vi "Miniquads.IDQuery.vi"(0 "i ref in":refnum<vi>, 3 "ms timeout (10000)":i32=10000, 5 "error in (no error)":errorcluster) -> (14 "i ref out":refnum<vi>, 15 "DeviceID":string, 17 "timed out":bool, 19 "error out":errorcluster)   [LabVIEW 2014, in "Miniquads.lvlib"]
doc: "Gets and sets the device ID."
uses:
  Miniquads.lvlib
  CS_Core/CSSystem/CSSystemLib/CSSystemLib.lvlib
  CSlibraries-extern/DimLVEvent/NodeMon-LV/LVNodeInfo/LVNodeInfo.lvlib
  CS_Core/CSApplicationBaseClasses/DeviceBase/DeviceBase.lvlib
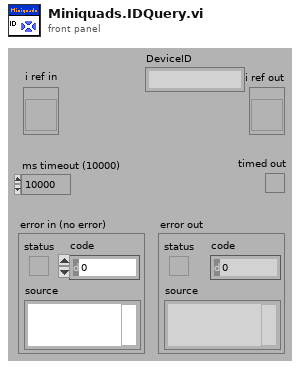
[diagram p1: front panel]
types:
  T1 = cluster{"Major":u16, "Minor":u16, "Fix":u16, "Build":u16}
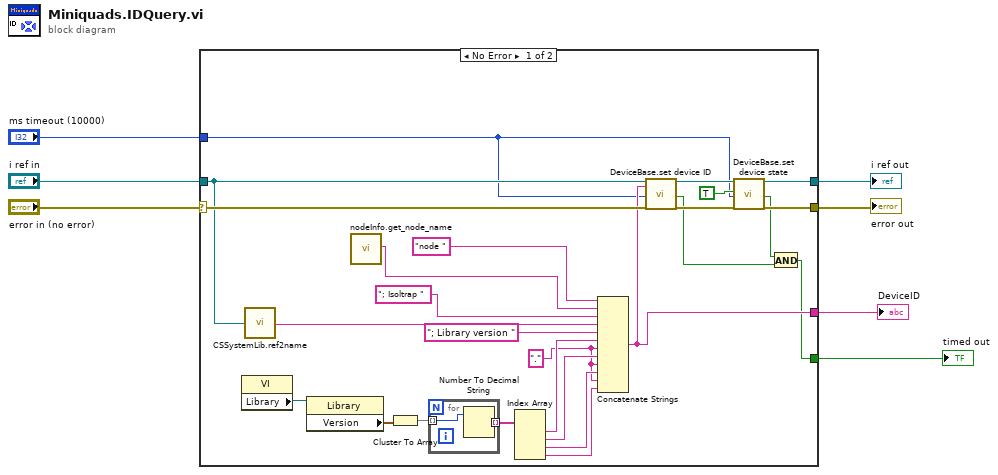
[diagram p0: block diagram]
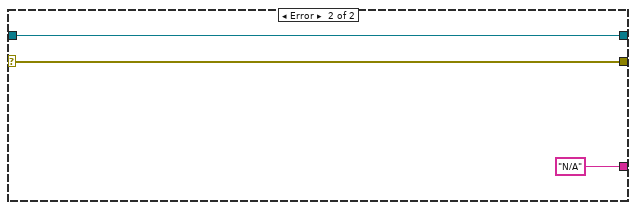
[diagram p2: hidden frame]
diagram:
  n1 = case shown="No Error" "error in (no error)" {
    selector: "error in (no error)" -> [w30 w37]
    tunnel: "i ref in" -> [w22 w38]
    tunnel: [w31 w38] -> w6
    tunnel: [w28 w37] -> w5
    tunnel: "ms timeout (10000)" -> [w11 _]
    tunnel: [w23 "N/A"] -> w2
    tunnel: [w8 _] -> w1
    frame No Error {
      w12 = "."
      n2 = property class="VI"() -> ("Library"=w21:refnum<vi>)  [unwired: 2 in, 2 out]
      n3 = call "CSSystemLib.ref2name.vi"("obj refnum"=w22) -> ("name"=w24:string)
      n4 = property class="Library"(reference=w21) -> ("Version"=w20:T1)  [unwired: 1 in, 2 out]
      n5 = call "nodeInfo.get_node_name.vi"() -> ("nodeName"=w26:string)  [unwired: 18 in, 1 out]
      n6 = Cluster To Array(cluster=w20) -> (array=w19:u16[])
      n7 = for {
        tunnel: w19 -> [w35] mode=indexing
        tunnel: [w34] -> w18 mode=indexing
        n8 = Number To Decimal String(number=w35) -> (decimal integer string=w34:string)  [unwired: 1 in]
      }
      n9 = Index Array(array=w18) -> (element #1=w16:string, element #2=w15:string, element #3=w14:string, element #4=w13:string)  [unwired: 4 in]
      n10 = Concatenate Strings("node " ("string"), w26, "; Isoltrap ", w24, "; Library version " ("string"), w16, w12, w15, w12, w14, w12, w13) -> (w23:string)
      n11 = call "DeviceBase.set device ID.vi"("i ref in"=w22, "deviceID"=w23, "ms timeout (10000)"=w11, "error in (no error)"=w30) -> ("i ref out"=w32:refnum<vi>, "timed out"=w9:bool, "error out"=w29:errorcluster)  [unwired: 13 in]
      n12 = call "DeviceBase.set device state.vi"("i ref in"=w32, "implicit"=TRUE, "ms timeout (10000)"=w11, "error in (no error)"=w29) -> ("i ref out"=w31:refnum<vi>, "timed out"=w10:bool, "error out"=w28:errorcluster)  [unwired: 13 in]
      n13 = And(x=w10, y=w9) -> (x .and. y?=w8:bool)
    }
    frame Error {
    }
  }
  "error out" <- w5
  "i ref out" <- w6
  "timed out" <- w1
  "DeviceID" <- w2
